vi "CE XCL Write header.vi"(6 "AC source idn":string, 7 "Digitizer idn":string, 8 "error in (no error)":errorcluster, 11 "CE measurement":T1={"Signal frequencies (Hz) T"=[1000.0], "Signal amplitudes (V) T"=[0.707], "Sampling frequencies (Hz) T"=[10000000.0], "Record lengths (multiples of periods) T"=[10000.0], "TWM data root directory"=path "", "TWM mreasurements directories"=[], "Calculate RMS from samples"=FALSE, "Algorithm to use"="TWM-WFFT", "Quantity to read"="TWM-WFFT", "Settle down after AC source change (s) T"=1.0, "Skip PJVS setup"=FALSE, "Measurement template file"=path "", "Row of START keyword T"=0, "Row of STOP keyword T"=0, "Measurement template line T"=[], "Switch position T"=[10000.0], "FR fit mat file T"=path "", "Recalculate-skip already calculated"=FALSE} {"Switch position T" format="%#_3p"; "Record lengths (multiples of periods) T" format="%#_3p"; "Sampling frequencies (Hz) T" format="%#_3p"; "Signal amplitudes (V) T" format="%#_3p"; "Signal frequencies (Hz) T" format="%#_3p"}) -> (0 "error out":errorcluster, 5 "NI_report out":refnum<class "NI_report.lvclass">)   [LabVIEW 2020]
doc: "Writes devices identifications into CE template."
uses:
  <vilib>/Utility/NIReport.llb/NI_report.lvclass
  CE Measurement/Type definitions/CE measurement.ctl
  <vilib>/Utility/NIReport.llb/Report Type.ctl
  <vilib>/Utility/NIReport.llb/NI_ReportGenerationCore.lvlib
  external libraries/varilib/varilib.lvlib
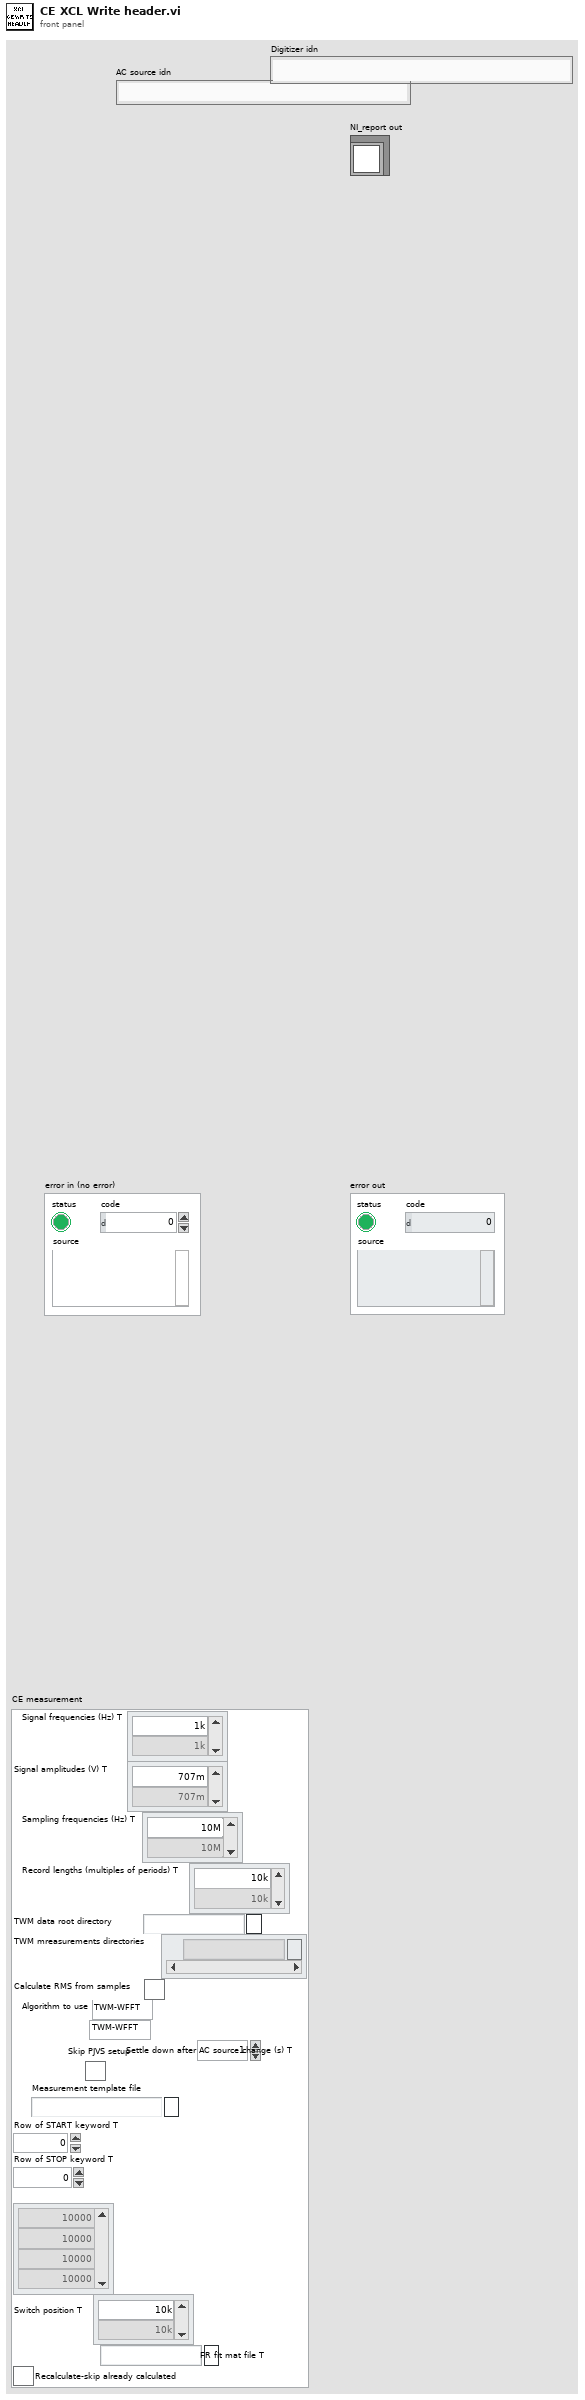
[diagram p1: front panel]
types:
  T1 = typedef "CE measurement.ctl" = cluster{"Signal frequencies (Hz) T":dbl[], "Signal amplitudes (V) T":dbl[], "Sampling frequencies (Hz) T":dbl[], "Record lengths (multiples of periods) T":dbl[], "TWM data root directory":path, "TWM mreasurements directories":path[], "Calculate RMS from samples":bool, "Algorithm to use":string, "Quantity to read":string, "Settle down after AC source change (s) T":dbl, "Skip PJVS setup":bool, "Measurement template file":path, "Row of START keyword T":i32, "Row of STOP keyword T":i32, "Measurement template line T":i32[], "Switch position T":dbl[], "FR fit mat file T":path, "Recalculate-skip already calculated":bool}
  T2 = enum16{"maximized", "minimized", "normal", "no change"}
  T3 = typedef "NI_ReportGenerationCore.lvlib/Report Type.ctl" = enum16{"HTML", "Word", "Excel"}
  T4 = typedef "Type definitions to be saved.ctl" = cluster{"Common properties":T5, "AC Source":T6, "DC meter":T8, "CE measurement":T1, "FR measurement":T10, "FR template":T11, "CE template":T12, "PJVS":T13, "SS measurement":T17, "AC sync source":T6, "DG measurement":T18}
  T5 = typedef "Common properties.ctl" = cluster{"Measurement status ref":refnum<vi>, "TWM Status ref":refnum<vi>, "Abort ref":refnum<vi>, "Skip waiting ref":refnum<vi>, "GNU Octave path":path, "TWM+QWTB path":path, "lvlib path":path, "TWM pipe":string, "PJVS status ref":refnum<vi>, "WAC path":path}
  T6 = typedef "AC Source.ctl" = cluster{"AC Source type":T7, "VISA":refnum<visa-resource-name>, "Ref. clock (Hz)":dbl, "status ref":refnum<vi>, "Fluke 57XX wideband output":bool, "Fluke 57XX ignore errors":bool, "Synchronization by AC signal":bool}
  T7 = typedef "AC Source type.ctl" = enum16{"Fluke 5XXX calibrator", "Tektronix AFG3000 series", "dummy", "Agilent 331xxA to 332xxA", "Agilent 335xxA to 336xxA"}
  T8 = typedef "DC meter.ctl" = cluster{"DC meter type":T9, "DC meter VISA":refnum<visa-resource-name>, "NPLC":dbl, "status ref":refnum<vi>}
  T9 = typedef "DC meter type.ctl" = enum16{"H/A/K 3458", "Fluke 8508A", "dummy", "Keithley 2182"}
  T10 = typedef "FR measuement.ctl" = cluster{"Measurement frequencies (Hz)":dbl[], "Sampling frequency (Hz)":dbl, "Signal amplitude (V)":dbl, "AC-DC settle time (s)":dbl, "Record length (multiples of period)":dbl[], "Measurement template file":path, "Row of START keyword":i32, "Row of STOP keyword":i32, "Calculate RMS from samples":bool, "AC-DC warm up time (s)":dbl, "Measurement template line":i32[], "DC meter readings No.":i32, "Algorithm":string, "Simultaneous measurement":bool, "Recalculate-skip already calculated":bool}
  T11 = typedef "FR template.ctl" = cluster{"Keywords column":i32, "Sig. freq. column":i32, "Rec. len. column":i32, "Meas. points. row min to read":i32, "Meas. points. row max to read":i32, "Properties column":i32, "Properties row start":i32, "Properties row end":i32, "Keyword START regexp":string, "Keyword STOP regexp":string, "HW data column":i32, "HW data row start":i32, "HW data row end":i32, "TIme and date column start":i32, "Digitizer value column start ":i32, "DC mean column start ":i32, "DC readings column start":i32}
  T12 = typedef "CE template.ctl" = cluster{"Keywords column":i32, "Sig. freq. column":i32, "Rec. len. column":i32, "Switch pos column":i32, "Meas. points. row min to read":i32, "Meas. points. row max to read":i32, "Properties column":i32, "Properties row start":i32, "Properties row end":i32, "Keyword START regexp":string, "Keyword STOP regexp":string, "HW data column":i32, "HW data row start":i32, "HW data row end":i32, "TIme and date column start":i32, "Digitizer value column start ":i32}
  T13 = typedef "PJVS.ctl" = cluster{"PJVS type":T14, "Status Refnum":refnum<vi>, "AC-supraVOLTcontrol":cluster{"IP address:port (0.0.0.0:0000)":string, "Timeouts":T15, "Simulation mode":bool, "Debug mode":bool}, "NPL bias source":cluster{"DataSocketCluster":T16}, "Manual PJVS":cluster{"PJVS frequency (Hz)":dbl, "Reference voltages (V)":dbl[], "File with PJVS voltages":path}, "VTT PJVS":cluster{"some VTT only property":string}}
  T14 = typedef "PJVS Type.ctl" = enum16{"AC-supraVOLTcontrol", "JV modified NPL bias control", "Manual PJVS", "VTT PJVS"}
  T15 = typedef "ACSVcontrol-driver.lvlib/Timeouts.ctl" = cluster{"TCP Read & Write (ms)":i32, "Sensors readout":i32, "PJVS setup":i32, "Nullmeter readout":i32, "Multiplexer setup":i32, "57XX setup":i32, "Generator setup":i32, "Synthesizer setup":i32, "Sampler readout":i32}
  T16 = typedef "DataSocketCluster external.ctl" = cluster{"Server Machine":string, "Client Machine":string, "Data":string, "TimeStamp":dbl, "Count":i32, "Target Process":string}
  T17 = typedef "SS measurement.ctl" = cluster{"Signal frequencies (Hz)":dbl[], "Signal amplitudes (V)":dbl[], "Sampling frequencies (Hz)":dbl[], "Record lengths (multiples of periods)":dbl[], "Calculate results":bool, "Algorithm":string, "TWM data directories":path[], "TWM data directories relative":path[], "Settle down after AC source change (s)":dbl, "PJVS frequencies (Hz)":dbl[], "PJVS reference voltages array of vector cluster":cluster{"PJVS reference voltages vector":dbl[]}[], "Requested PJVS steps":u32[], "Measure CE":bool, "Measure CE before":bool, "Measure CE after":bool, "Single point CE measurement":bool, "original CE template path":path, "new CE template path before SS":path, "new CE template path before SS relative":path, "new CE template path after SS":path, "new CE template path after SS relative":path, "original CE fit path":path, "new CE fit path before SS":path, "new CE fit path before SS relative":path, "new CE fit path after SS":path, "new CE fit path after SS relative":path, "Measure digitizer gain":bool, "Measure digitizer gain before":bool, "Measure digitizer gain after":bool, "Digitizer gain":dbl, "Data folder":path, "FR fit path":path, "new FR fit path relative":path, "Rs":i32, "Re":i32, "SS measurement info files":path[]}
  T18 = typedef "DG measurement.ctl" = cluster{"Sampling frequencies (Hz)":dbl[], "Requested PJVS frequencies (Hz)":dbl[], "Requested PJVS waveform amplitudes (V)":dbl[], "Record lengths (multiples of PJVS periods)":dbl[], "Requested PJVS steps":u32[], "Switch position":dbl, "Settle down after PJVS change (s)":dbl, "Rs":i32, "Re":i32, "Algorithm":string, "Calculate results":bool, "Data folder":path, "TWM data directories":path[], "TWM data directories relative":path[], "DG measurement info files":path[], "Set PJVS frequencies (Hz)":dbl[], "Set PJVS reference voltages array of vector cluster":cluster{"PJVS reference voltages vector":dbl[]}[], "Set PJVS steps":u32[]}
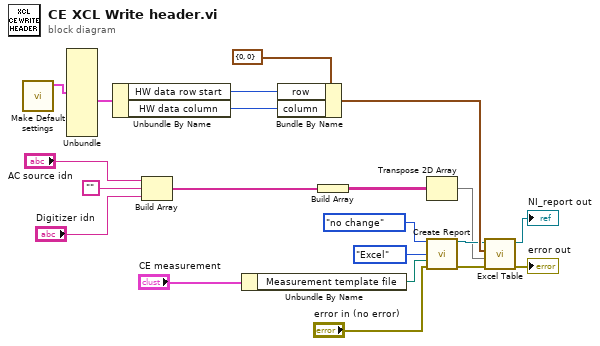
[diagram p0: block diagram]
diagram:
  n1 = call "Make Default settings.vi"() -> ("TD to be saved"=w6:T4)  [unwired: 11 in]
  n2 = Unbundle(w6) -> ("CE template"=w3:T12)  [unwired: 10 out]
  n3 = Unbundle By Name(w3) -> ("HW data row start"=w5:i32, "HW data column"=w4:i32)
  n4 = Build Array("AC source idn", "", "Digitizer idn") -> (w15:string[])
  n5 = Unbundle By Name("CE measurement") -> ("Measurement template file"=w7:path)
  n6 = Bundle By Name(cluster=cluster{"row":i32, "column":i32} {"row"=0, "column"=0} ("start (0, 0)"), "row"=w5, "column"=w4) -> (w17:cluster{"row":i32, "column":i32})
  n7 = Build Array(w15) -> (w10:string[][])
  n8 = Transpose 2D Array(2D array=w10) -> (transposed array=w9:string[][])
  n9 = call <vilib>:"Create Report.vi"("window state (normal)"=T2."no change", "report type"=Report_Type."Excel", "template (empty)"=w7, "error in (no error)"="error in (no error)") -> ("report out"=w12:refnum<class "NI_report.lvclass">, "error out"=w14:errorcluster)  [unwired: 10 in]
  n10 = call "Excel Table.vi"("error in (no error)"=w14, "table"=w9, "start (0, 0)"=w17, "report in"=w12) -> ("error out"=→"error out":errorcluster, "report out"=→"NI_report out":refnum<class "NI_report.lvclass">)  [unwired: 6 in]
